vi "MF-101 Industrial Digital Input - Voltage Threshold.vi"() -> ()   [LabVIEW 8.6]
uses:
  <libdir>/resource/objmgr/ueidaq.rc
  vi.lib/UeiDaq/UeiDaqConfigureTimingForSimpleIO.vi
  vi.lib/UeiDaq/UeiDaqReadOneScaledScan.vi
  vi.lib/UeiDaq/UeiDaqCreateDIIndustrialSession.vi
  vi.lib/UeiDaq/UeiDaqReadOneDigitalScanUInt16.vi
panel:
  out "DI Resolution":u32
  out "Diagnostic  data ( volts )":dbl[](array[numeric]) format="%#_4g"
  in  "Diagnostic Resource":string
  in  "stop":bool
  in  "in range":bool[](array[boolean])
  in  "High threshhold":dbl[](array[numeric]) caption="(digital input on at this voltage, max =55V )"
  in  "Low threshold":dbl[](array[numeric]) caption="(digital input off at this voltage, min = 0V)"
  out "Device":string
  out "High Threshhold read":dbl[](array[numeric])
  out "Low Threshhold read":dbl[](array[numeric])
  in  "Digital Input Resource":string
  # "MF-101 Industrial Digital Input - Voltage Threshold"
  # "1/ Set the resource name -->"
  # "pdna://192.168.100.2/dev0/di0/0\npdna://192.168.100.2/dev0/diline0:15"
  # "0"
  # "1"
  # "2"
  # "3"
  # "4"
  # "5"
  # "6"
  # "7"
  # "8"
  # "9"
  # "10"
  # "11"
  # "12"
  # "13"
  # "14"
  # "15"
  # "diag ch        name\n     8            adc_fet0\n     9            adc_fet1\n   10            adc_fet2\n   11            adc_fet3\n   12            adc_fet4\n   13            adc_fet5\n   14            adc_fet6\n   15            adc_fet7\n   16            adc_fet8\n   17            adc_fet9\n   18           adc_fet10\n   19           adc_fet11\n   20           adc_fet12\n   21           adc_fet13\n   22           adc_fet14\n   23           adc_fet15"
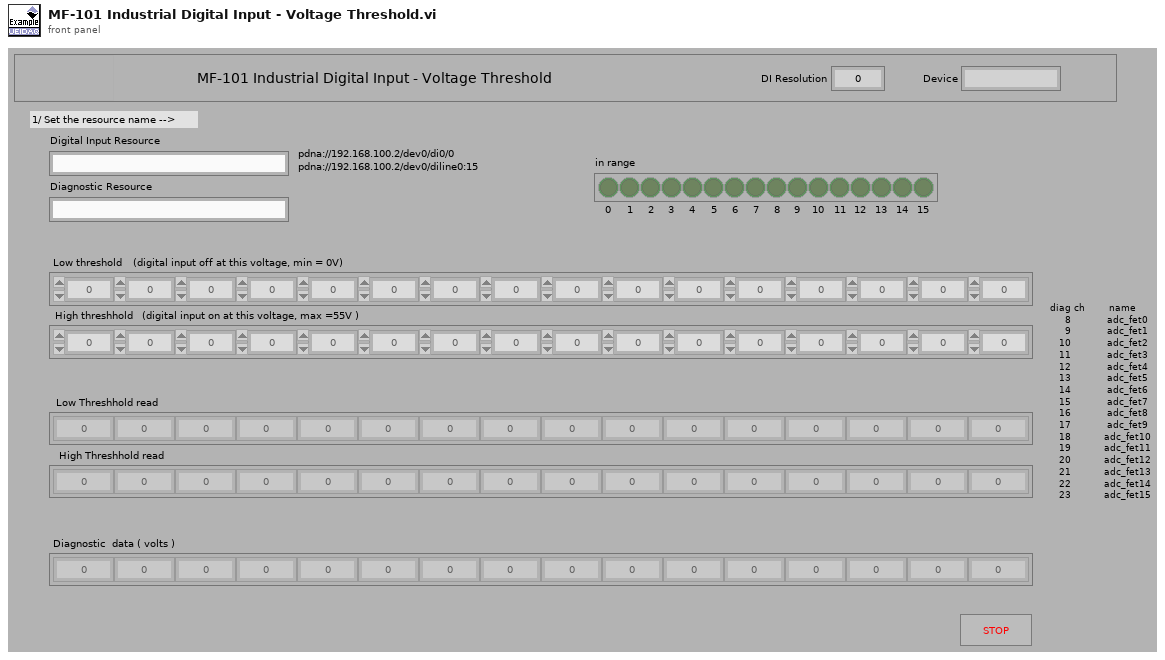
[diagram p1: front panel]
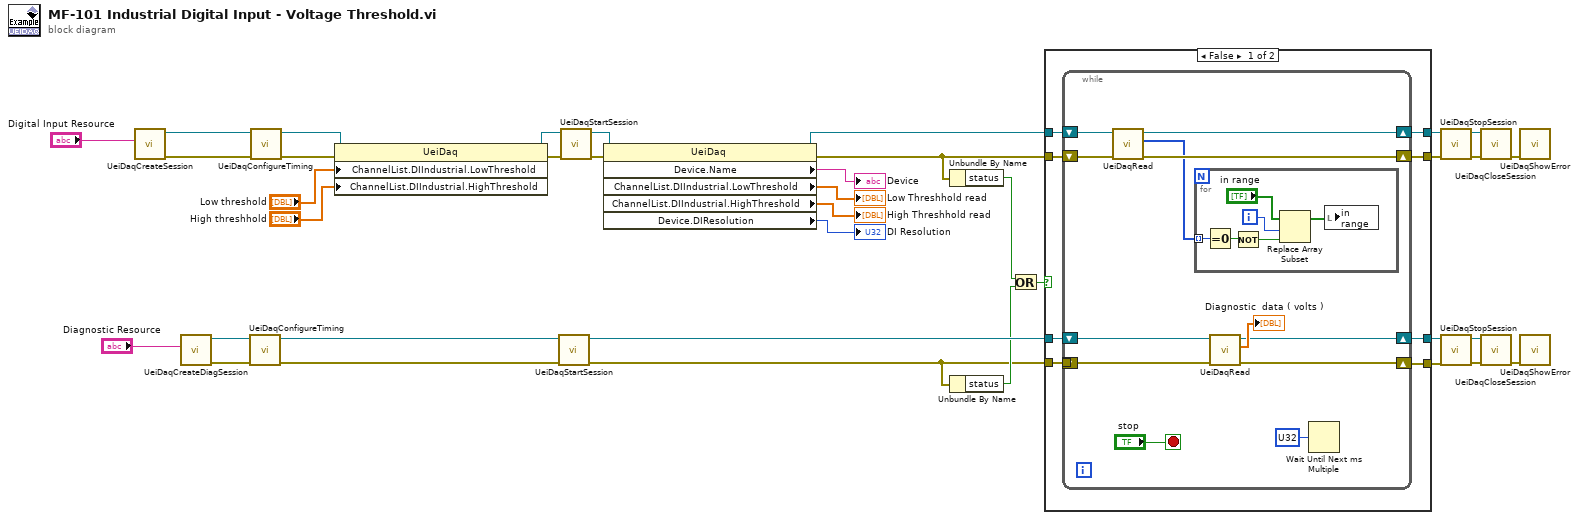
[diagram p0: block diagram]
diagram:
  n1 = call-poly "UeiDaqCreateSession.vi"("Resource"="Digital Input Resource") -> ("error out"=w35:errorcluster, "UeiDaq Refnum Out"=w36:refnum<k20>)  [unwired: 6 in, 3 out]
  n2 = call "UeiDaqCreateDiagSession.vi"("Resource"="Diagnostic Resource") -> ("error out"=w15:errorcluster, "UeiDaq Refnum Out"=w16:refnum<k20>)  [unwired: 9 in]
  n3 = call-poly "UeiDaqConfigureTiming.vi"("error in (no error)"=w15, "UeiDaq Refnum In"=w16) -> ("error out"=w17:errorcluster, "UeiDaq Refnum Out"=w18:refnum<k20>)  [unwired: 8 out]
  n4 = call-poly "UeiDaqConfigureTiming.vi"("error in (no error)"=w35, "UeiDaq Refnum In"=w36) -> ("error out"=w31:errorcluster, "UeiDaq Refnum Out"=w32:refnum<k20>)  [unwired: 1 in, 7 out]
  n5 = property class="UeiDaq"(reference=w32, error in=w31, "ChannelList.DIIndustrial.LowThreshold"="Low threshold", "ChannelList.DIIndustrial.HighThreshold"="High threshhold") -> (reference out=w28:refnum<k20>, error out=w27:errorcluster)
  n6 = call "UeiDaqStartSession.vi"("error in (no error)"=w17, "UeiDaq Refnum In"=w18) -> ("error out"=w10:errorcluster, "UeiDaq Refnum Out"=w13:refnum<k20>)  [unwired: 8 in]
  n7 = call "UeiDaqStartSession.vi"("error in (no error)"=w27, "UeiDaq Refnum In"=w28) -> ("error out"=w26:errorcluster, "UeiDaq Refnum Out"=w25:refnum<k20>)  [unwired: 8 in]
  n8 = property class="UeiDaq"(reference=w25, error in=w26) -> (reference out=w20:refnum<k20>, error out=w19:errorcluster, "Device.Name"=→"Device":string, "ChannelList.DIIndustrial.LowThreshold"=→"Low Threshhold read":dbl[], "ChannelList.DIIndustrial.HighThreshold"=→"High Threshhold read":dbl[], "Device.DIResolution"=→"DI Resolution":u32)
  n9 = Unbundle By Name(w19) -> ("status"=w12:bool)
  n10 = Unbundle By Name(w10) -> ("status"=w11:bool)
  n11 = Or(x=w12, y=w11) -> (x .or. y?=w9:bool)
  n12 = case shown="False" w9 {
    tunnel: w20 -> [w45 w67]
    tunnel: w19 -> [w44 w66]
    tunnel: [w43 w67] -> w23
    tunnel: [w42 w66] -> w22
    tunnel: w13 -> [w41 w65]
    tunnel: w10 -> [w40 w64]
    tunnel: [w39 w65] -> w5
    tunnel: [w38 w64] -> w4
    frame #0 {
      n13 = while {
        shift-right: [w55] -> w43
        shift-left: w45 -> [w57]
        shift-right: [w54] -> w42
        shift-left: w44 -> [w56]
        tunnel: w40 -> [w50]
        shift-right: [w49] -> w39
        shift-left: w41 -> [w51]
        shift-right: [w48] -> w38
        shift-left: _ -> [_]
        stop <- "stop" stop-if-true
        n14 = call-poly "UeiDaqRead.vi"("error in (no error)"=w56, "UeiDaq Refnum In"=w57) -> ("error out"=w54:errorcluster, "Raw Data"=w46:i16[], "UeiDaq Refnum Out"=w55:refnum<k20>)  [unwired: 7 in]
        n15 = for {
          tunnel: w46 -> [w63] mode=indexing
          i -> [w62]
          n16 = Equal To 0?(x=w63) -> (x = 0?=w61:bool)
          n17 = Not(x=w61) -> (.not. x?=w60:bool)
          n18 = Replace Array Subset(array="in range", new element=w60, index=w62) -> (w58:bool[])
          n19 = local write "in range"(w58) -> ()
        }
        n20 = call-poly "UeiDaqRead.vi"("error in (no error)"=w50, "UeiDaq Refnum In"=w51) -> ("error out"=w48:errorcluster, "Scaled Data"=→"Diagnostic  data ( volts )":dbl[], "UeiDaq Refnum Out"=w49:refnum<k20>)  [unwired: 7 in]
        n21 = Wait Until Next ms Multiple(millisecond multiple=u32 ?) -> ()  [unwired: 1 out]
      }
    }
    frame #1 {
    }
  }
  n22 = call "UeiDaqStopSession.vi"("error in (no error)"=w22, "UeiDaq Refnum In"=w23) -> ("error out"=w29:errorcluster, "UeiDaq Refnum Out"=w30:refnum<k20>)  [unwired: 8 in]
  n23 = call "UeiDaqStopSession.vi"("error in (no error)"=w4, "UeiDaq Refnum In"=w5) -> ("error out"=w8:errorcluster, "UeiDaq Refnum Out"=w7:refnum<k20>)  [unwired: 8 in]
  n24 = call "UeiDaqCloseSession.vi"("error in (no error)"=w29, "UeiDaq Refnum In"=w30) -> ("error out"=w37:errorcluster)  [unwired: 1 in, 8 out]
  n25 = call "UeiDaqCloseSession.vi"("error in (no error)"=w8, "UeiDaq Refnum In"=w7) -> ("error out"=w6:errorcluster)  [unwired: 1 in, 8 out]
  n26 = call "UeiDaqShowError.vi"("error in (no error)"=w37) -> ()  [unwired: 2 in, 9 out]
  n27 = call "UeiDaqShowError.vi"("error in (no error)"=w6) -> ()  [unwired: 2 in, 9 out]
